vi "Is_Valid_VI.vi"(8 "error in (no error)":errorcluster, 10 "standardVI? (T)":bool=TRUE, 11 "AB_Source_VI in":refnum<class "AB_Source_VI.lvclass">) -> (0 "error out":errorcluster, 1 "PDC":bool, 2 "VI":bool, 3 "AB_Source_VI out":refnum<class "AB_Source_VI.lvclass">)   [LabVIEW 2020, in "AB_Source_VI.lvclass"]
uses:
  <vilib>/AppBuilder/AB_Classes/Source/VI/AB_Source_VI.lvclass
  <vilib>/AppBuilder/AB_Classes/Source/VI/AB_Source_VI.lvclass/AB_Source_VI.ctl
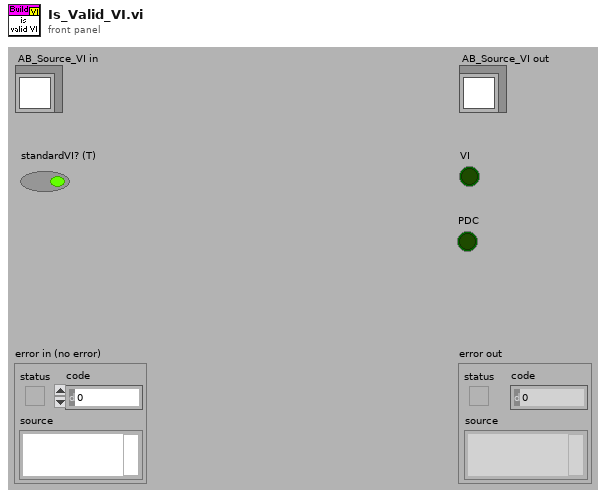
[diagram p1: front panel]
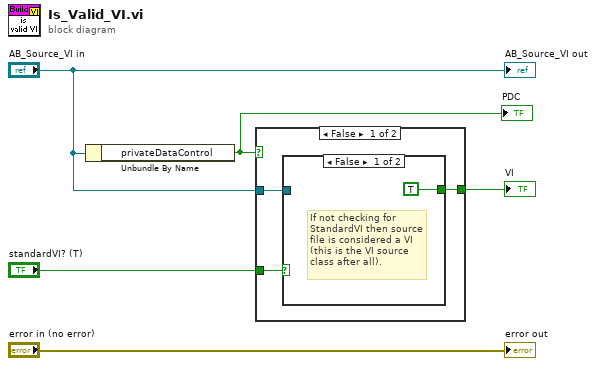
[diagram p0: block diagram]
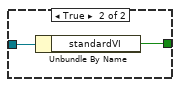
[diagram p2: hidden frame]
diagram:
  n1 = Unbundle By Name("AB_Source_VI in") -> ("privateDataControl"=w1:bool)
  "PDC" <- w1
  n2 = case shown="False" w1 {
    tunnel: [w8 _] -> w4
    tunnel: "AB_Source_VI in" -> [w7 _]
    tunnel: "standardVI? (T)" -> [w6 _]
    frame False {
      n3 = case shown="False" w6 {
        tunnel: [TRUE ("standardVI") w11] -> w8
        tunnel: w7 -> [_ w10]
        frame False {
          # "If not checking for StandardVI then source file is considered a VI (this is the VI source class after all)."
        }
        frame True {
          n4 = Unbundle By Name(w10) -> ("standardVI"=w11:bool)
        }
      }
    }
    frame True {
      # "When adding files to a build, a PDC is not a valid VI file."
    }
  }
  "VI" <- w4
  "error out" <- "error in (no error)"
  "AB_Source_VI out" <- "AB_Source_VI in"
